vi "test_5772_stage1.vi"() -> ()   [LabVIEW 2013]
uses:
  <vilib>/measure/maspectr.llb/Power Spectrum and PSD Export Mode.ctl
  <vilib>/measure/maspectr.llb/FFT Power Spectrum and PSD for 1 Chan (CDB).vi
  <vilib>/measure/NI_MAPro.lvlib
panel:
  out "Waveform Graph 2":i16[](graph)
  out "size before":i32
  out "Waveform Graph":dbl[](graph)
  out "power spectrum":cluster{"f0":dbl, "df":dbl, "magnitude":dbl[]}(graph)
  out "size after":i32
  out "Q out":fxp<+/-,16,14>[](array[numeric])
  out "I out":fxp<+/-,16,14>[](array[numeric])
  out "iteration1":i32
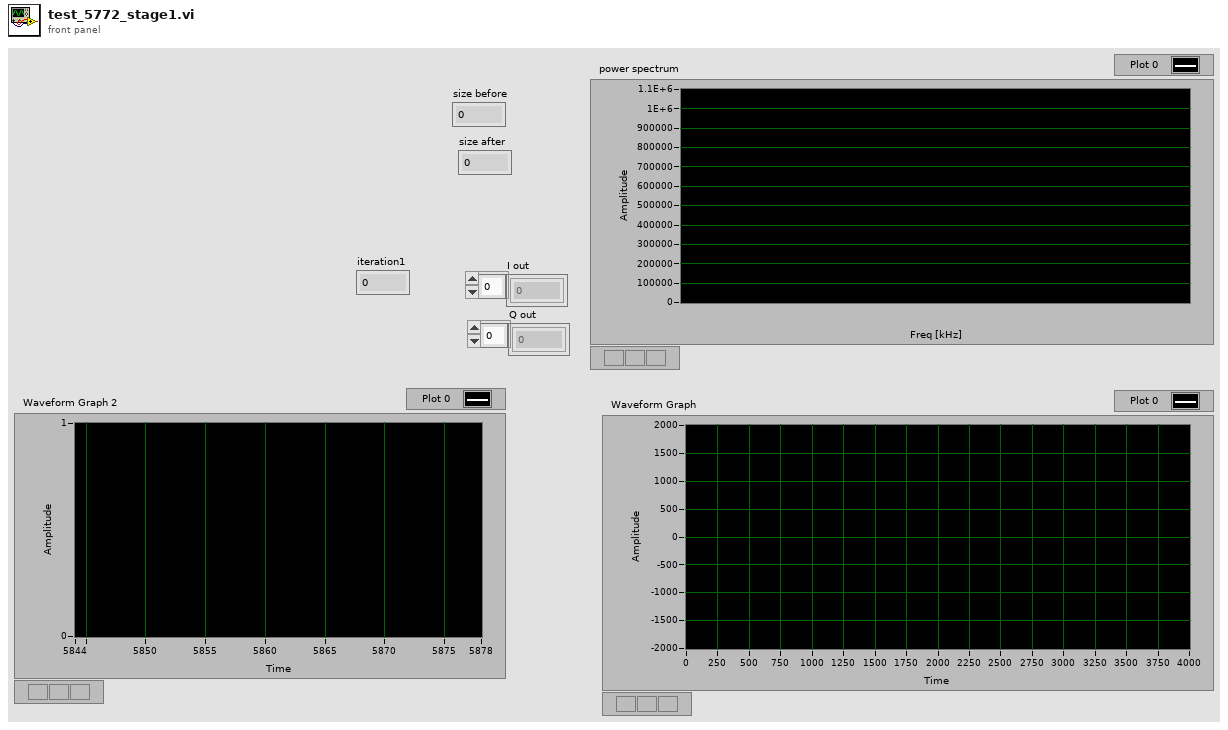
[diagram p1: front panel]
types:
  T1 = typedef "NI_MAPro.lvlib/Power Spectrum and PSD Export Mode.ctl" = u16
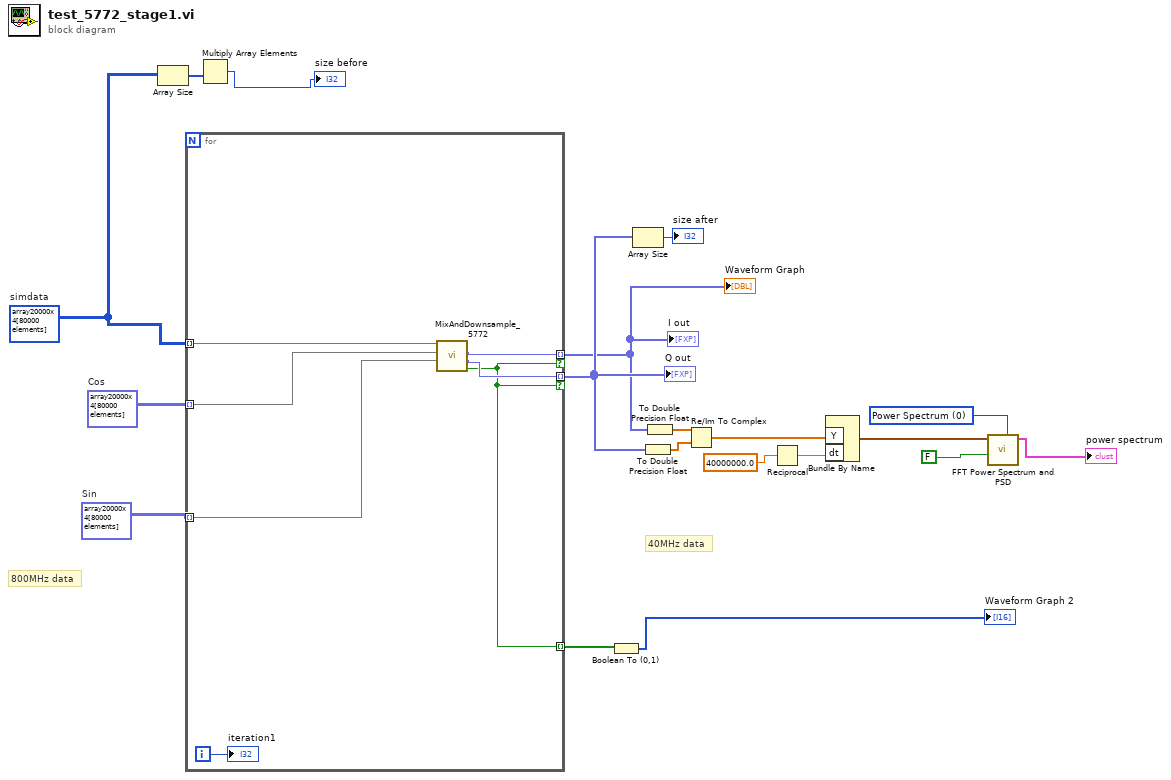
[diagram p0: block diagram]
diagram:
  w8 = fxp<+/-,16,0>[][] array20000x4[80000 elements]  # Cos
  w9 = i16[][] array20000x4[80000 elements]  # simdata
  w7 = fxp<+/-,16,0>[][] array20000x4[80000 elements]  # Sin
  w18 = T1 0 items=["Power Spectrum", "Power Spectral Density"] ("export mode")
  # "40MHz data"
  # "800MHz data"
  n1 = Array Size(array=w9) -> (size(s)=w4:i32[])
  n2 = for {
    tunnel: [w22] -> w5 mode=indexing if=w20
    tunnel: [w21] -> w6 mode=indexing if=w20
    tunnel: w9 -> [w25] mode=indexing
    tunnel: w7 -> [w24] mode=indexing
    tunnel: w8 -> [w23] mode=indexing
    tunnel: [w20] -> w2 mode=indexing
    i -> [w26]
    n3 = call "MixAndDownsample_5772.vi"("Sine in"=w24, "Cosine in"=w23, "Signal Input"=w25) -> ("data valid"=w20:bool, "Q out"=w21:fxp<+/-,16,14>, "I out"=w22:fxp<+/-,16,14>)  [unwired: 6 in]
    "iteration1" <- w26
  }
  "I out" <- w5
  "Q out" <- w6
  "Waveform Graph" <- w5
  n4 = Multiply Array Elements(1:w4) -> (0:→"size before":i32)
  n5 = Boolean To (0,1)(Boolean=w2) -> (0, 1=→"Waveform Graph 2":i16[])
  n6 = Array Size(array=w6) -> (size(s)=→"size after":i32)
  n7 = To Double Precision Float(number=w6) -> (double precision float=w11:dbl[])
  n8 = To Double Precision Float(number=w5) -> (double precision float=w12:dbl[])
  n9 = Re/Im To Complex(1:w11, 2:w12) -> (0:w10:cdb[])
  n10 = Reciprocal(x=40000000.0 ("dt")) -> (1/x=w14:dbl)
  n11 = Bundle By Name("Y"=w10, "dt"=w14) -> (w17:waveform(cdb))  [unwired: 1 in]
  n12 = call-poly <vilib>:"FFT Power Spectrum and PSD.vi"("export mode"=w18, "dB On (F)"=FALSE, "time signal"=w17) -> ("Power Spectrum / PSD"=→"power spectrum":cluster{"f0":dbl, "df":dbl, "magnitude":dbl[]})  [unwired: 5 in, 3 out]
